vi "Set Path Control - Value and Enabled.vi"(8 "error in (no error)":errorcluster, 9 "Value":path, 10 "Enabled?":bool, 11 "Path in":refnum<vi>) -> (0 "error out":errorcluster)   [LabVIEW 2014, in "RIO Target.lvclass"]
uses:
  RIO Target.lvclass
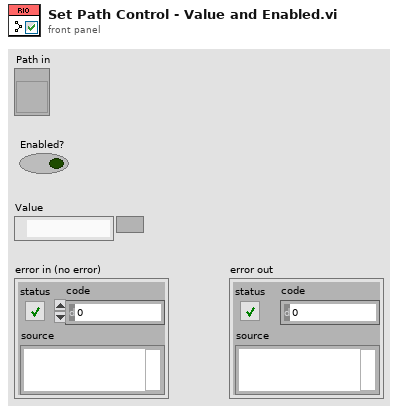
[diagram p1: front panel]
types:
  T1 = enum8{"Enabled", "Disabled", "Disabled and Grayed Out"}
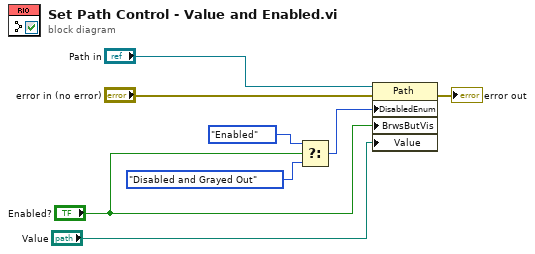
[diagram p0: block diagram]
diagram:
  n1 = Select(t=T1."Enabled" ("Disabled"), s="Enabled?", f=T1."Disabled and Grayed Out" ("Disabled")) -> (s? t:f=w8:T1)
  n2 = property class="Path"(reference="Path in", error in="error in (no error)", "DisabledEnum"=w8, "BrwsButVis"="Enabled?", "Value"="Value") -> (error out=→"error out":errorcluster)  [unwired: 1 out]
